vi "Perform_Meas_Setup.vi"(2 "Simulate/Run":T1, 3 "String array":string[](array[string])) -> (0 "Continue?":bool)   [LabVIEW 2013]
uses:
  Controls/User_Specific_mode.ctl
  Controls/Setup.ctl
  Controls/Save_Data.ctl
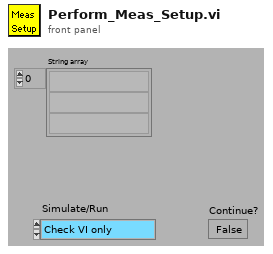
[diagram p1: front panel]
types:
  T1 = typedef "User_Specific_mode.ctl" = enum16{"Check VI only", "Run VI"}
  T2 = typedef "Save_Data.ctl" = enum16{"Save No Data", "Save Data"}
  T3 = typedef "Setup.ctl" = enum16{"Run Program", "Show Setup", "Save Current Setup", "Setup Front Panel"}
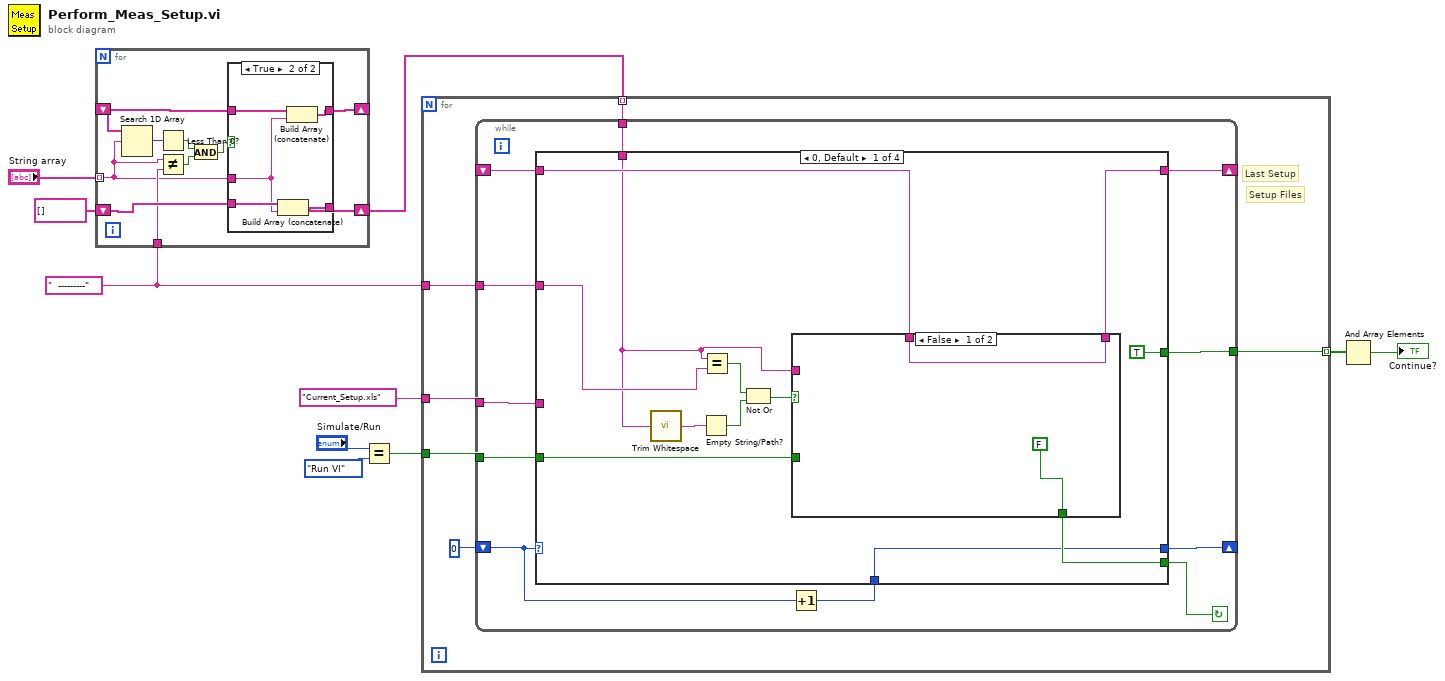
[diagram p0: block diagram]
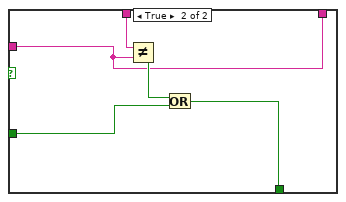
[diagram p3: hidden frame]
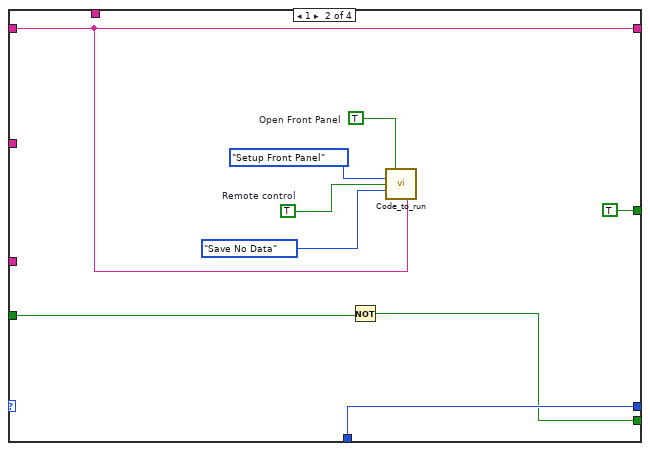
[diagram p4: hidden frame]
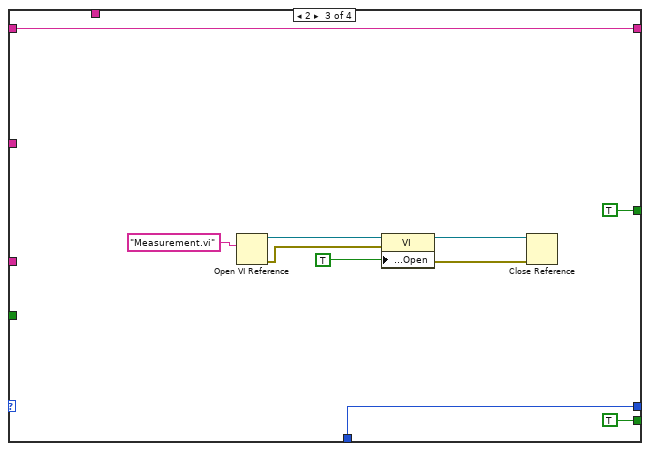
[diagram p5: hidden frame]
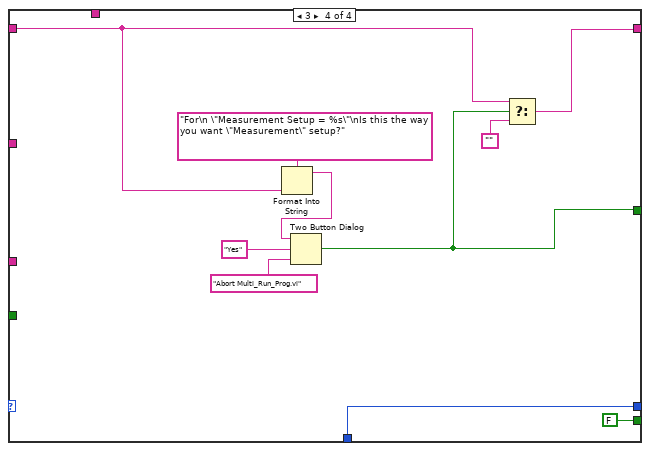
[diagram p6: hidden frame]
diagram:
  w1 = "  ---------" ("f")
  n1 = for {
    shift-right: [w19] -> _
    shift-left: _ -> [w20]
    shift-right: [w17] -> w2
    shift-left: string[] [] -> [w18]
    tunnel: "String array" -> [w14] mode=indexing
    tunnel: w1 -> [w15]
    n2 = Search 1D Array(1D array=w20, element=w14) -> (index of element=w16:i32)  [unwired: 1 in]
    n3 = Less Than 0?(x=w16) -> (x < 0?=w11:bool)
    n4 = Not Equal?(x=w14, y=w15) -> (x != y?=w12:bool)
    n5 = And(x=w11, y=w12) -> (x .and. y?=w13:bool)
    n6 = case shown="True" w13 {
      tunnel: w14 -> [_ w23]
      tunnel: w20 -> [w22 w27]
      tunnel: [w22 w26] -> w19
      tunnel: w18 -> [w21 w25]
      tunnel: [w21 w24] -> w17
      frame False {
      }
      frame True {
        n7 = Build Array (concatenate)(w25, w23) -> (w24:string[])
        n8 = Build Array (concatenate)(w27, w23) -> (w26:string[])
      }
    }
  }
  n9 = Equal?(x="Simulate/Run", y=User_Specific_mode."Run VI" ("Simulate/Run")) -> (x = y?=w7:bool)
  n10 = for {
    tunnel: "Current_Setup.xls" ("name or relative path") -> [w32]
    tunnel: w7 -> [w31]
    tunnel: w2 -> [w30] mode=indexing
    tunnel: [w29] -> w6 mode=indexing
    tunnel: w1 -> [w28]
    # "Last Setup"
    # "Setup Files"
    n11 = while {
      tunnel: w31 -> [w36]
      tunnel: w32 -> [w37]
      shift-left: _ -> [w39]
      shift-right: [w38] -> _
      tunnel: [w40] -> w29
      shift-left: 0 -> [w43]
      shift-right: [w41] -> _
      tunnel: w30 -> [w35]
      tunnel: w28 -> [w34]
      stop <- w44 continue-if-true
      n12 = Increment(x=w43) -> (x+1=w42:i32)
      n13 = case shown="0, Default" w43 {
        tunnel: [w53 w67 TRUE FALSE] -> w44
        tunnel: w42 -> [w51 w69 w82 w92]
        tunnel: [w51 w69 w82 w92] -> w41
        tunnel: [TRUE ("T button?") TRUE ("T button?") TRUE ("T button?") w86] -> w40
        tunnel: w39 -> [w55 w64 w81 w84]
        tunnel: [w54 w64 w81 w85] -> w38
        tunnel: w37 -> [_ _ _ _]
        tunnel: w36 -> [w52 w68 _ _]
        tunnel: w35 -> [w46 _ _ _]
        tunnel: w34 -> [w47 _ _ _]
        frame 0, Default {
          n14 = call <vilib>:"Trim Whitespace.vi"("string"=w46) -> ("trimmed string"=w45:string)  [unwired: 1 in]
          n15 = Empty String/Path?(string/path=w45) -> (empty?=w49:bool)
          n16 = Equal?(x=w46, y=w47) -> (x = y?=w50:bool)
          n17 = Not Or(1:w49, 2:w50) -> (0:w48:bool)
          n18 = case shown="False" w48 {
            tunnel: [w58 w60] -> w54
            tunnel: w46 -> [_ w60]
            tunnel: w55 -> [w58 w63]
            tunnel: [FALSE w61] -> w53
            tunnel: w52 -> [_ w59]
            frame False {
            }
            frame True {
              n19 = Not Equal?(x=w63, y=w60) -> (x != y?=w62:bool)
              n20 = Or(x=w62, y=w59) -> (x .or. y?=w61:bool)
            }
          }
        }
        frame 1 {
          w71 = TRUE  # Remote control
          w72 = TRUE  # Open Front Panel
          n21 = Not(x=w68) -> (.not. x?=w67:bool)
          n22 = call "Code_to_run.vi"("Open Front Panel"=w72, "setup"=Setup."Setup Front Panel", "Remote control"=w71, "File"=Save_Data."Save No Data", "Setup filename"=w64) -> ()  [unwired: 5 in, 6 out]
        }
        frame 2 {
          n23 = Open VI Reference(vi path="Measurement.vi") -> (vi reference=w77:refnum<vi>, error out=w78:errorcluster)  [unwired: 1 in, 4 out]
          n24 = property class="VI"(reference=w77, error in=w78, "Front Panel Window:Open"=TRUE) -> (reference out=w75:refnum<vi>, error out=w74:errorcluster)
          n25 = Close Reference(reference=w75, error in (no error)=w74) -> ()  [unwired: 1 out]
        }
        frame 3 {
          n26 = Format Into String(format string="For\n \"Measurement Setup = %s\"\nIs this the way you want \"Measurement\" setup?" ("message"), w84) -> (resulting string=w91:string)  [unwired: 2 in, 1 out]
          n27 = Two Button Dialog(message=w91, 1:"Abort Multi_Run_Prog.vi" ("F button name (\"Cancel\")"), 2:"Yes" ("T button name (\"OK\")")) -> (T button?=w86:bool)
          n28 = Select(t=w84, s=w86, f="") -> (s? t:f=w85:string)
        }
      }
    }
  }
  n29 = And Array Elements(Boolean array=w6) -> (logical AND=→"Continue?":bool)
